vi "Average Amp (SubVI).vi"(10 "Numeric":i32, 11 "Array in":cluster{dbl, "y":dbl}[](array[cluster])) -> (2 "x/y":dbl, 3 "Array out":cluster{dbl, dbl}[](array[cluster]))   [LabVIEW 2017]
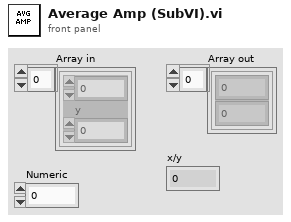
[diagram p1: front panel]
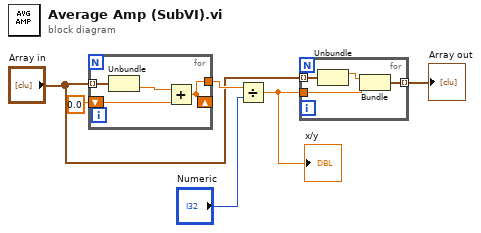
[diagram p0: block diagram]
diagram:
  n1 = for {
    tunnel: "Array in" -> [w10] mode=indexing
    shift-right: [w7] -> _
    shift-left: 0.0 -> [w8]
    tunnel: [w7] -> w5
    n2 = Unbundle(w10) -> ("y"=w9:dbl)  [unwired: 1 out]
    n3 = Add(x=w9, y=w8) -> (x+y=w7:dbl)
  }
  n4 = Divide(x=w5, y="Numeric") -> (x/y=w3:dbl)
  "x/y" <- w3
  n5 = for {
    tunnel: w3 -> [w13]
    tunnel: "Array in" -> [w14] mode=indexing
    tunnel: [w11] -> w1 mode=indexing
    n6 = Unbundle(w14) -> (w12:dbl)  [unwired: 1 out]
    n7 = Bundle(w12, w13) -> (w11:cluster{dbl, dbl})  [unwired: 1 in]
  }
  "Array out" <- w1
